vi "Data Generator_Create.vi"(0 "reference in":refnum<class "Data Generator.lvclass">, 11 "Error In":errorcluster) -> (4 "reference out":refnum<class "Data Generator.lvclass">, 15 "Error Out":errorcluster)   [LabVIEW 2024, in "Data Generator.lvclass"]
uses:
  Data Generator.lvclass
panel:
  # "Connector Pane"
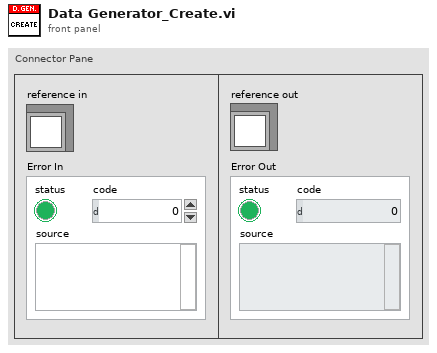
[diagram p1: front panel]
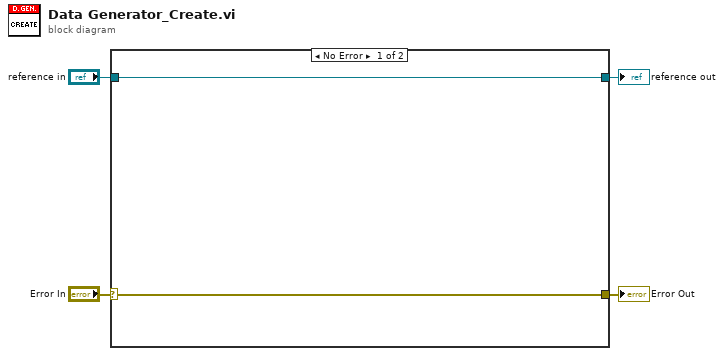
[diagram p0: block diagram]
diagram:
  n1 = case shown="No Error" "Error In" {
    selector: "Error In" -> [w5 w8]
    tunnel: [w5 w8] -> w3
    tunnel: "reference in" -> [w6 w7]
    tunnel: [w6 w7] -> w1
    frame No Error {
    }
    frame Error {
      # "VI-TechBaseTemplate_Simple_4x4x4"
    }
  }
  "Error Out" <- w3
  "reference out" <- w1
